vi "ExpUpdateParameter.vi"(8 "error in (no error)":errorcluster, 9 "Name (empty)":string, 10 "Variant":variant, 11 "ExpID":string) -> (0 "error out":errorcluster)   [LabVIEW 2017]
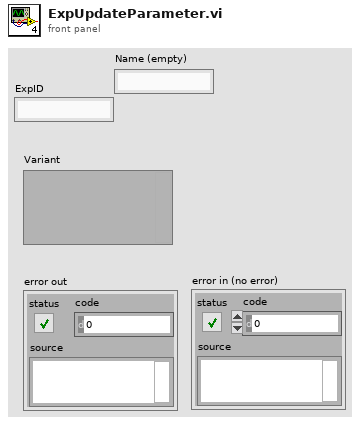
[diagram p1: front panel]
types:
  T1 = typedef "ExperimentInfo.ctl" = cluster{"ExposeInfo":T2, "ExpID":string, "ExperimentFilename":string}
  T2 = typedef "ExposeInfo.ctl" = cluster{"CSCom":refnum<k24>, "URL":string, "Events Category":string, "ID":string}
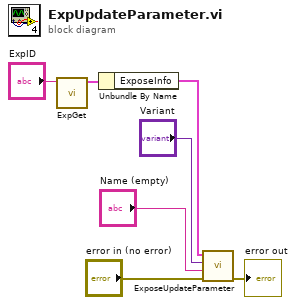
[diagram p0: block diagram]
diagram:
  n1 = call "ExpGet.vi"("ExpID"="ExpID") -> ("Exp Info"=w5:T1)  [unwired: 10 in]
  n2 = Unbundle By Name(w5) -> ("ExposeInfo"=w6:T2)
  n3 = call "ExposeUpdateParameter.vi"("error in (no error)"="error in (no error)", "Name (empty)"="Name (empty)", "Parameter"="Variant", "Expose Info"=w6) -> ("error out"=→"error out":errorcluster)  [unwired: 7 in]
